vi "SaveOnly.vi"(8 "error in (no error)":errorcluster, 10 "Path":path, 11 "Preferences in":refnum<class "SetListPrefs.lvclass">) -> (0 "error out":errorcluster, 2 "XML out":string, 3 "Preferences out":refnum<class "SetListPrefs.lvclass">)   [LabVIEW 2013, in "SetListPrefs.lvclass"]
uses:
  SetListPrefs.lvclass
panel:
  # "Leave Path Deafult as EMPTY PATH"
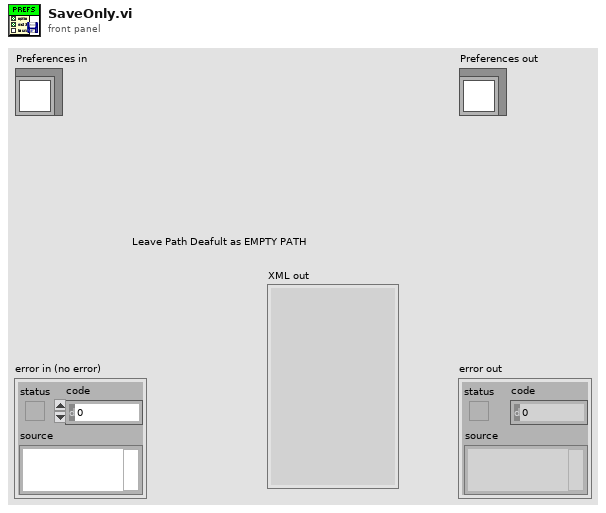
[diagram p1: front panel]
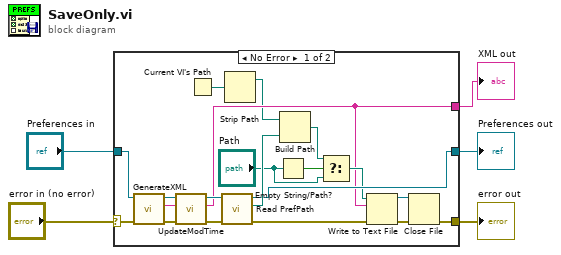
[diagram p0: block diagram]
diagram:
  n1 = case shown="No Error" "error in (no error)" {
    selector: "error in (no error)" -> [w24 w27]
    tunnel: [w19 w27] -> w4
    tunnel: [w18 w26] -> w2
    tunnel: "Preferences in" -> [w25 w26]
    tunnel: [w8 _] -> w1
    frame No Error {
      n2 = call "GenerateXML.vi"("error in (no error)"=w24, "Preferences in"=w25) -> ("error out"=w15:errorcluster, "FullXML"=w16:string, "Preferences out"=w14:refnum<class "SetListPrefs.lvclass">)  [unwired: 7 in]
      n3 = call "UpdateModTime.vi"("error in (no error)"=w15, "XML in"=w16, "Preferences in"=w14) -> ("error out"=w17:errorcluster, "XML out"=w8:string, "Preferences out"=w13:refnum<class "SetListPrefs.lvclass">)  [unwired: 6 in]
      n4 = Current VI's Path() -> (path=w7:path)
      n5 = call-dynamic "Read PrefPath.vi"("error in (no error)"=w17, "Preferences in"=w13) -> ("error out"=w22:errorcluster, "PrefPath"=w23:path, "Preferences out"=w18:refnum<class "SetListPrefs.lvclass">)  [unwired: 7 in]
      n6 = Strip Path(path=w7) -> (stripped path=w6:path)  [unwired: 1 out]
      n7 = Empty String/Path?(string/path="Path") -> (empty?=w12:bool)
      n8 = Build Path(base path=w6, name or relative path=w23) -> (appended path=w11:path)
      n9 = Select(t=w11, s=w12, f="Path") -> (s? t:f=w9:path)
      n10 = Write to Text File(file (use dialog)=w9, text=w8, error in=w22) -> (refnum out=w20:refnum<file>, error out=w21:errorcluster)  [unwired: 1 in, 1 out]
      n11 = Close File(refnum=w20, error in=w21) -> (error out=w19:errorcluster)  [unwired: 1 out]
    }
    frame Error {
    }
  }
  "error out" <- w4
  "Preferences out" <- w2
  "XML out" <- w1
